vi "arrays.vi"() -> ()   [LabVIEW 2013]
panel:
  out "Child 2 Final":i16[](array[numeric])
  out "Child 1 Final":i16[](array[numeric])
  out "array (last n elements first) 2":i32[](array[numeric])
  out "Shuffled Array":i32[](array[numeric])
  out "array (last n elements first)":i32[](array[numeric])
  out "array w/ subset deleted":i32[](array[numeric])
  out "output array":i32[](array[numeric])
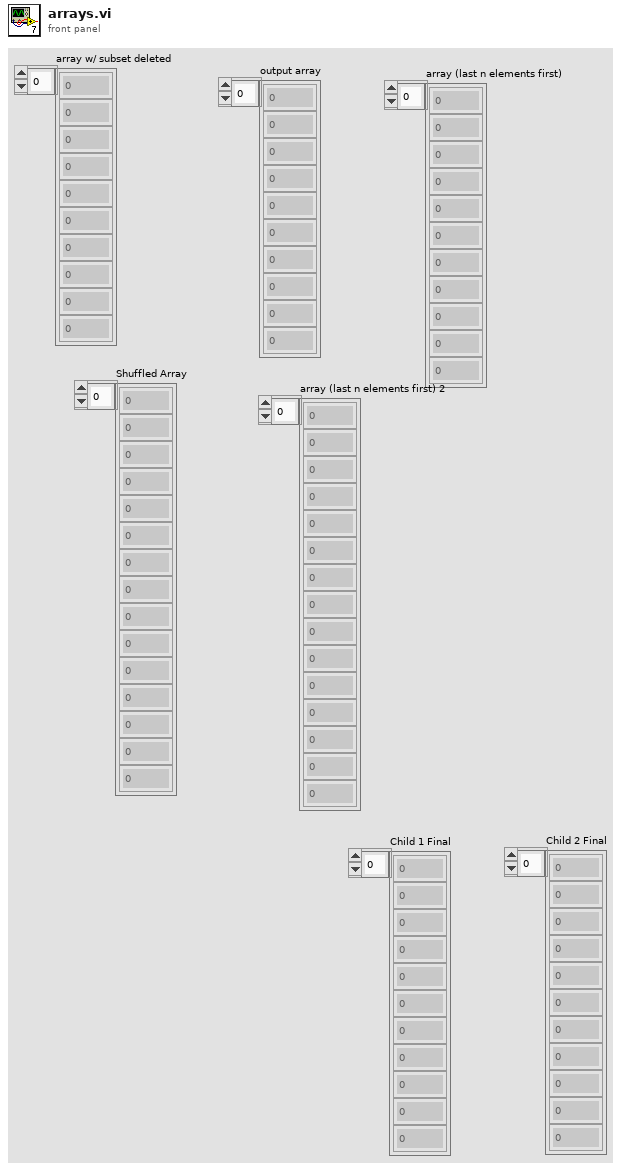
[diagram p1: front panel]
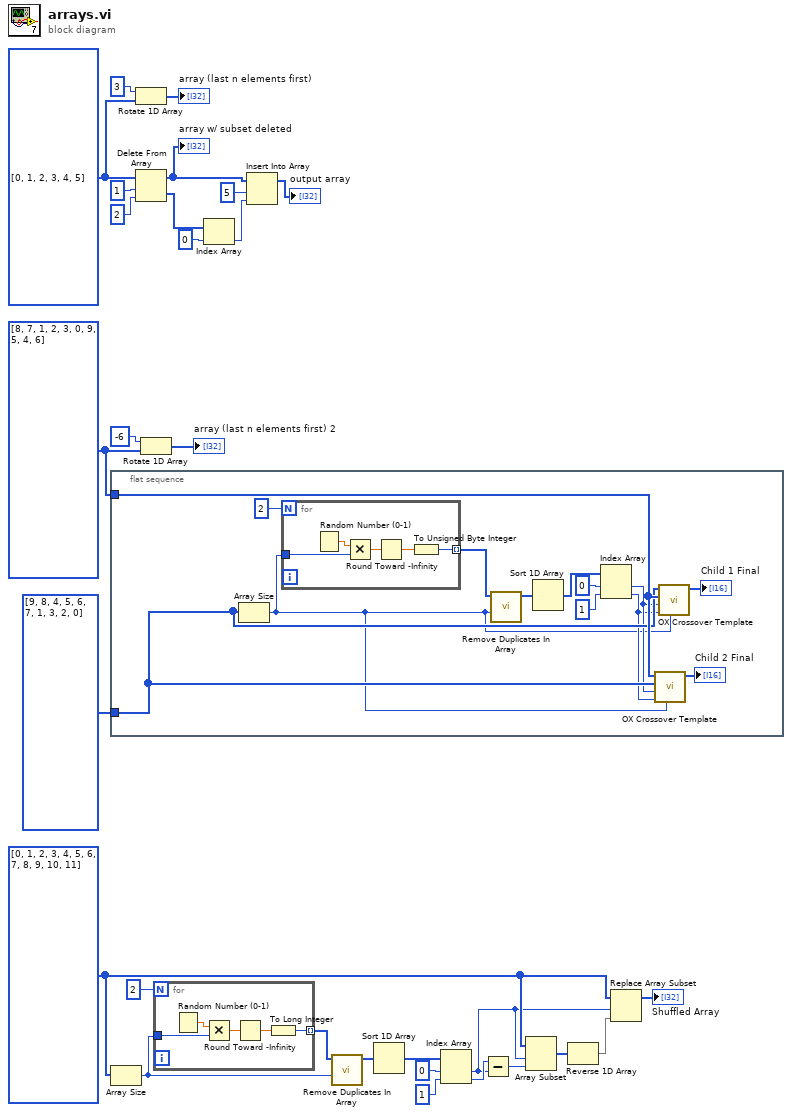
[diagram p0: block diagram]
diagram:
  w1 = u16[] [8, 7, 1, 2, 3, 0, 9, 5, 4, 6]
  w18 = i32[] [0, 1, 2, 3, 4, 5, 6, 7, 8, 9, 10, 11]
  w21 = i32[] [0, 1, 2, 3, 4, 5]
  n1 = flat-sequence {
    tunnel: u16[] [9, 8, 4, 5, 6, 7, 1, 3, 2, 0] ("Schedule") -> [w34]
    tunnel: w1 -> [w35]
    frame #0 {
      n2 = Array Size(array=w34) -> (size(s)=w31:i32)
      n3 = for {
        N: 2 -> [_]
        tunnel: w31 -> [w46]
        tunnel: [w43] -> w41 mode=indexing
        n4 = Random Number (0-1)() -> (number: 0 to 1=w47:dbl)
        n5 = Multiply(x=w47, y=w46) -> (x*y=w45:dbl)
        n6 = Round Toward -Infinity(1:w45) -> (0:w44:dbl)
        n7 = To Unsigned Byte Integer(number=w44) -> (unsigned 8bit integer=w43:u8)
      }
      n8 = call "Remove Duplicates In Array.vi"("Max Index Bound"=w31, "Random Numbers Array"=w41) -> ("Random Numbers Array without Duplicates"=w40:i32[])  [unwired: 9 in]
      n9 = Sort 1D Array(array=w40) -> (sorted array=w39:i32[])
      n10 = Index Array(array=w39, index #1=0 ("index"), index #2=1 ("index")) -> (element #1=w33:i32, element #2=w32:i32)
      n11 = call "OX Crossover Template.vi"("Array Size"=w31, "Index 2"=w32, "Index 1"=w33, "Schedule 2"=w34, "Schedule 1"=w35) -> ("Child"=→"Child 2 Final":u16[])  [unwired: 6 in]
      n12 = call "OX Crossover Template.vi"("Array Size"=w31, "Index 2"=w32, "Index 1"=w33, "Schedule 2"=w35, "Schedule 1"=w34) -> ("Child"=→"Child 1 Final":u16[])  [unwired: 6 in]
    }
  }
  n13 = Array Size(array=w18) -> (size(s)=w14:i32)
  n14 = Rotate 1D Array(1:w21, 2:3 ("n")) -> (0:→"array (last n elements first)":i32[])
  n15 = Delete From Array(array=w21, length=1, index=2) -> (deleted portion=w25:i32[], array with subset deleted=w22:i32[])
  "array w/ subset deleted" <- w22
  n16 = Rotate 1D Array(1:w1, 2:-6 ("n")) -> (0:→"array (last n elements first) 2":u16[])
  n17 = for {
    N: 2 -> [_]
    tunnel: w14 -> [w49]
    tunnel: [w48] -> w15 mode=indexing
    n18 = Random Number (0-1)() -> (number: 0 to 1=w52:dbl)
    n19 = Multiply(x=w52, y=w49) -> (x*y=w51:dbl)
    n20 = Round Toward -Infinity(1:w51) -> (0:w50:dbl)
    n21 = To Long Integer(number=w50) -> (32bit integer=w48:i32)
  }
  n22 = Index Array(array=w25, index=0) -> (element=w23:i32)
  n23 = Insert Into Array(array=w22, index=5, new element=w23) -> (→"output array":i32[])
  n24 = call "Remove Duplicates In Array.vi"("Max Index Bound"=w14, "Random Numbers Array"=w15) -> ("Random Numbers Array without Duplicates"=w11:i32[])  [unwired: 9 in]
  n25 = Sort 1D Array(array=w11) -> (sorted array=w10:i32[])
  n26 = Index Array(array=w10, index #1=0 ("index"), index #2=1 ("index")) -> (element #1=w8:i32, element #2=w9:i32)
  n27 = Subtract(x=w9, y=w8) -> (x-y=w7:i32)
  n28 = Array Subset(array=w18, index=w8, length=w7) -> (w6:i32[])
  n29 = Reverse 1D Array(array=w6) -> (reversed array=w5:i32[])
  n30 = Replace Array Subset(array=w18, new element=w5, index=w8) -> (→"Shuffled Array":i32[])
